vi "Send.vi"(8 "error in":errorcluster, 11 "Expedited Download Transfer in":refnum<class "Download Expedited Transfer.lvclass">) -> (0 "error out":errorcluster)   [LabVIEW 2020, in "CANopen.lvlib" / "SDO Manager.lvlib" / "Download Expedited Transfer.lvclass"]
uses:
  Download Expedited Transfer.lvclass
  HAL/Source/Interfaces/ICommunicate/ICommunicate.lvclass
  CANopen Message/CANopen Message.lvclass
  Download Expedited Transfer.lvclass/Download Expedited Transfer.ctl
  Typedefs/Function Code.ctl
  CANopen.lvlib
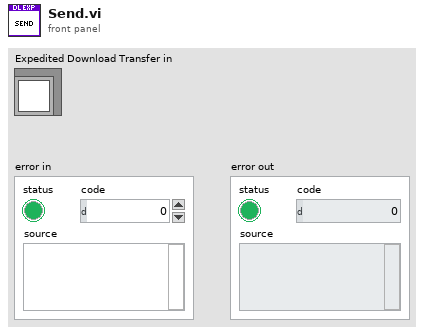
[diagram p1: front panel]
types:
  T1 = typedef "CANopen.lvlib/Function Code.ctl" = u8
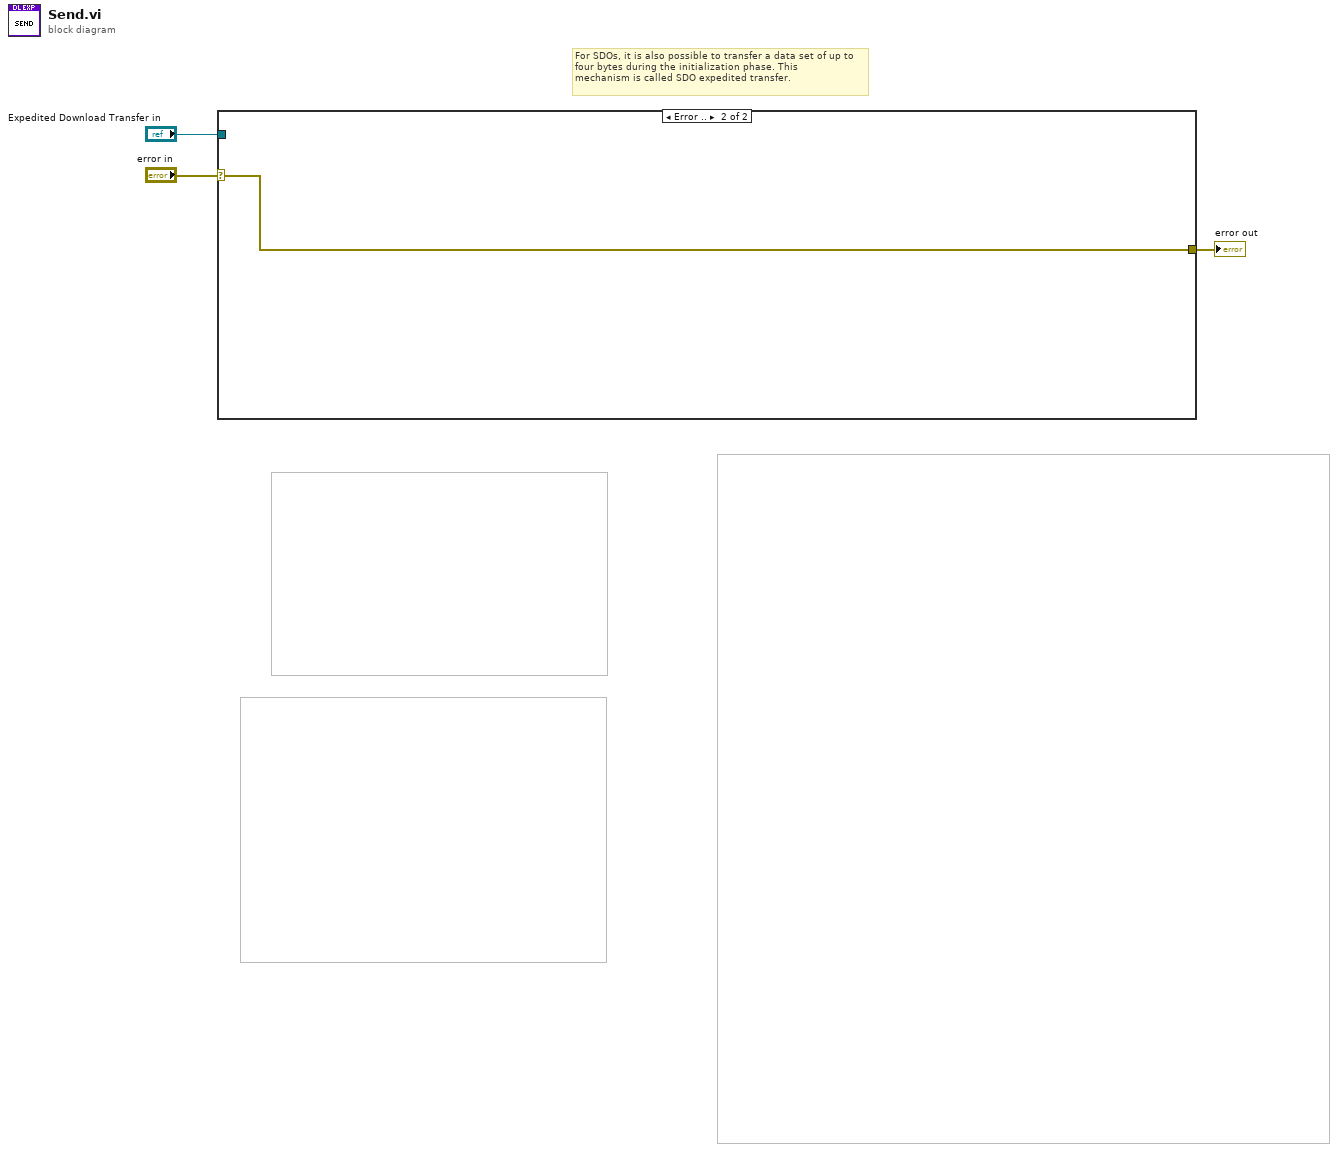
[diagram p0: block diagram]
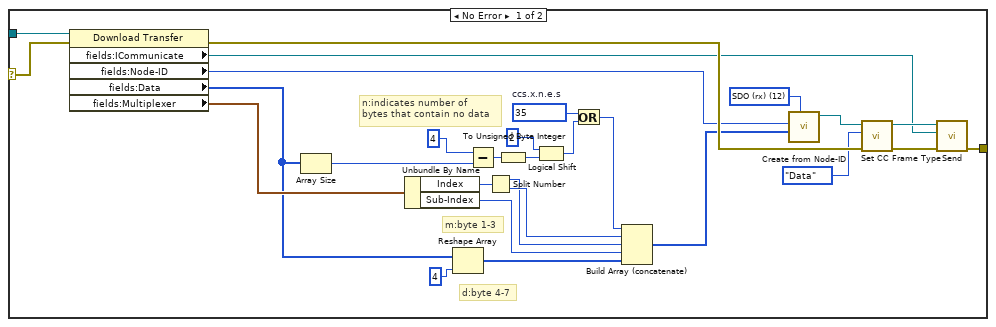
[diagram p2: hidden frame]
diagram:
  # "For SDOs, it is also possible to transfer a data set of up to four bytes during the initialization phase. This \nmechanism is called SDO expedited transfer."
  n1 = case shown="Error .." "error in" {
    selector: "error in" -> [w30 w32]
    tunnel: "Expedited Download Transfer in" -> [w29 _]
    tunnel: [w28 w32] -> w1
    frame No Error {
      w9 = T1 12 items=["NMT"=0, "EMCY/SYNC"=1, "TIME"=2, "PDO1 (tx)"=3, "PDO1 (rx)"=4, "PDO2 (tx)"=5, "PDO2 (rx)"=6, "PDO3 (tx)"=7, "PDO3 (rx)"=8, "PDO4 (tx)"=9, "PDO4 (rx)"=10, "SDO (tx)"=11, "SDO (rx)"=12, "NMT error control"=14] ("Function Code")
      w20 = u8 35  # ccs.x.n.e.s
      # "n:indicates number of\nbytes that contain no data"
      # "d:byte 4-7"
      # "m:byte 1-3"
      n2 = property class="Download Transfer"(reference=w29, error in=w30) -> (error out=w31:errorcluster, "fields:ICommunicate"=w4:refnum<class "ICommunicate.lvclass">, "fields:Node-ID"=w27:u8, "fields:Data"=w11:u8[], "fields:Multiplexer"=w13:cluster{"Index":u16, "Sub-Index":u8})  [unwired: 1 out]
      n3 = Array Size(array=w11) -> (size(s)=w12:i32)
      n4 = Unbundle By Name(w13) -> ("Index"=w26:u16, "Sub-Index"=w23:u8)
      n5 = Reshape Array(w11, 4 ("y")) -> (w19:u8[])
      n6 = Subtract(x=4 ("y"), y=w12) -> (x-y=w17:i32)
      n7 = Split Number(x=w26) -> (hi(x)=w24:u8, lo(x)=w25:u8)
      n8 = To Unsigned Byte Integer(number=w17) -> (unsigned 8bit integer=w16:u8)
      n9 = Logical Shift(y=i8 2, x=w16) -> (x << y=w15:u8)
      n10 = Or(x=w20, y=w15) -> (x .or. y?=w21:u8)
      n11 = Build Array (concatenate)(w21, w25, w24, w23, w19) -> (w10:u8[])
      n12 = call "Create from Node-ID.vi"("Function Code"=w9, "Data"=w10, "Node-ID"=w27) -> ("CANopen Message"=w8:refnum<class "CANopen Message.lvclass">)  [unwired: 8 in]
      n13 = call "Set CC Frame Type.vi"("error in"=w31, "CC Frame Type"=enum8{"Data", "Remote", "Error", "Overload"}."Data", "CANopen Message in"=w8) -> ("error out"=w7:errorcluster, "CANopen Message out"=w6:refnum<class "CANopen Message.lvclass">)  [unwired: 7 in]
      n14 = call "Send.vi"("error in"=w7, "ICommunicate"=w4, "CANopen Message in"=w6) -> ("error out"=w28:errorcluster)  [unwired: 7 in, 1 out]
    }
    frame Error {
    }
  }
  "error out" <- w1
